vi "chooseKickTo.vi"(0 "KickToSkill in":refnum<class "KickToSkill.lvclass">, 1 "Game in":refnum<class "Game.lvclass">, 8 "Robot":refnum<class "Robot.lvclass">, 9 "KickForce 0?":bool, 10 "use criteria?":bool=TRUE, 11 "ForceInGame":bool, 12 "BadDribblerIDs":i32[](array[numeric]), 13 "pass?":bool, 15 "firstCall":bool, 16 "ChipKickInEnemyField":bool, 17 "Target":dbl[](array[numeric])) -> (20 "Game out":refnum<class "Game.lvclass">, 21 "Robot out":refnum<class "Robot.lvclass">)   [LabVIEW 2020, in "ShootTactic.lvclass"]
uses:
  ShootTactic.lvclass
  KickToSkill_class/KickToSkill.lvclass
  Robot_class/robotKickToStates.ctl
  Robot_class/Robot.lvclass
  Game_class/Game.lvclass
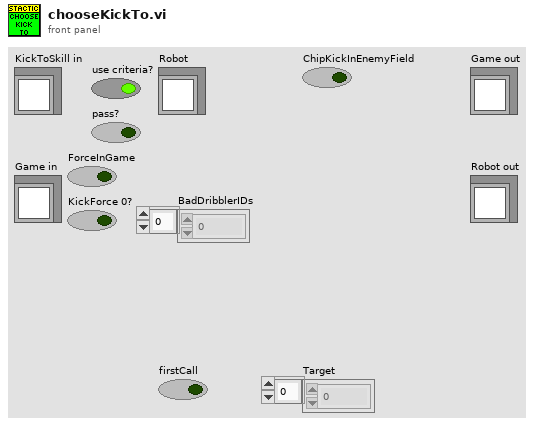
[diagram p1: front panel]
types:
  T1 = typedef "robotKickToStates.ctl" = enum16{"shootFromDirect", "avoidCollideBall", "goToBackBall", "none", "walk", "turn", "oldKickToShoot", "oldKickToGoToBackBall", "shoot"}
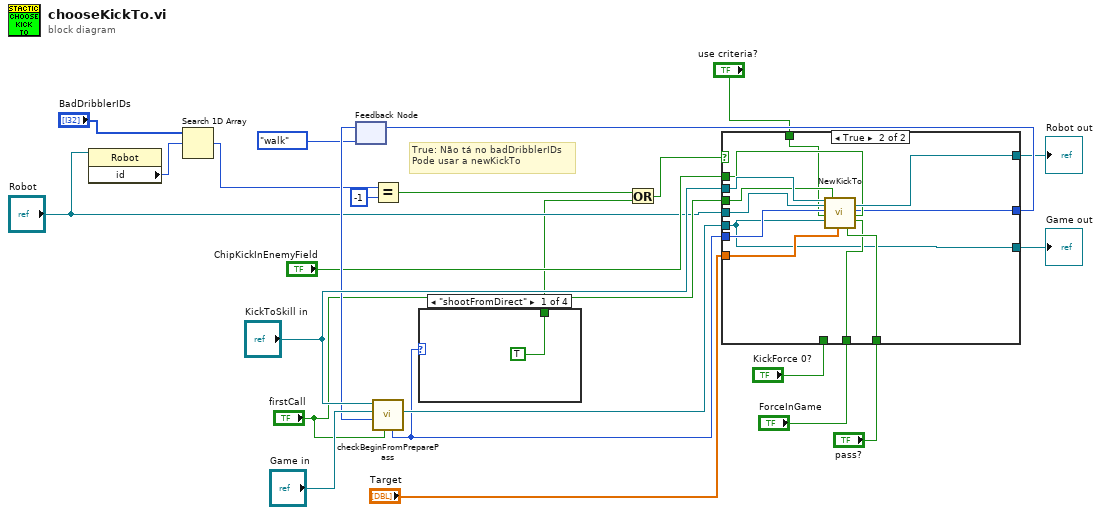
[diagram p0: block diagram]
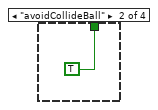
[diagram p2: hidden frame]
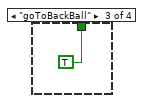
[diagram p3: hidden frame]
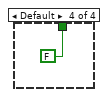
[diagram p4: hidden frame]
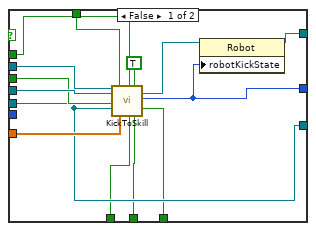
[diagram p5: hidden frame]
diagram:
  # "True: Não tá no badDribblerIDs\nPode usar a newKickTo"
  n1 = property class="Robot"(reference="Robot") -> ("id"=w7:i32)  [unwired: 1 in, 2 out]
  n2 = Search 1D Array(1D array="BadDribblerIDs", element=w7) -> (index of element=w6:i32)  [unwired: 1 in]
  n3 = feedback #1(robotKickToStates."walk" ("robotKickState")) -> (w20:T1)
  n4 = Equal?(x=w6, y=-1) -> (x = y?=w4:bool)
  n5 = call "checkBeginFromPreparePass.vi"("firstCall?"="firstCall", "robotKickState in"=w20, "Game in"="Game in", "KickToSkill in"="KickToSkill in") -> ("Game out"=w23:refnum<class "Game.lvclass">, "state out"=w3:T1)  [unwired: 3 in, 3 out]
  n6 = case shown="\"shootFromDirect\"" w3 {
    tunnel: [TRUE TRUE TRUE FALSE] -> w2
    frame "shootFromDirect" {
    }
    frame "avoidCollideBall" {
    }
    frame "goToBackBall" {
    }
    frame Default {
    }
  }
  n7 = Or(x=w4, y=w2) -> (x .or. y?=w5:bool)
  n8 = case shown="True" w5 {
    tunnel: "KickToSkill in" -> [w38 w54]
    tunnel: [w31 w53] -> w14
    tunnel: "Robot" -> [w42 w52]
    tunnel: "Target" -> [w40 w51]
    tunnel: w23 -> [w39 w43]
    tunnel: "firstCall" -> [w41 w50]
    tunnel: [w39 w43] -> w16
    tunnel: "ChipKickInEnemyField" -> [w37 w49]
    tunnel: w3 -> [_ w48]
    tunnel: [w30 w47] -> w24
    tunnel: "pass?" -> [w36 w45]
    tunnel: "ForceInGame" -> [w35 w44]
    tunnel: "KickForce 0?" -> [w34 _]
    tunnel: "use criteria?" -> [w33 w46]
    frame False {
      n9 = call "KickToSkill.vi"("KickToSkill in"=w38, "Robot"=w42, "firstCall?"=w41, "Game"=w39, "use criteria?"=w33, "Target"=w40, "chipKick ?"=w37, "KickForce 0?"=w34, "WeakKick"=TRUE, "ForceInGame"=w35, "pass?"=w36) -> ("Robot out"=w32:refnum<class "Robot.lvclass">, "robotKickState out"=w30:T1)  [unwired: 5 in, 2 out]
      n10 = property class="Robot"(reference=w32, "robotKickState"=w30) -> (reference out=w31:refnum<class "Robot.lvclass">)  [unwired: 1 in, 1 out]
    }
    frame True {
      n11 = call "NewKickTo.vi"("KickToSkill in"=w54, "Robot"=w52, "State in"=w48, "use criteria?"=w46, "Game"=w43, "firstCall?"=w50, "Target"=w51, "pass?"=w45, "chipKick ?"=w49, "ForceInGame"=w44) -> ("Robot out"=w53:refnum<class "Robot.lvclass">, "State out"=w47:T1)  [unwired: 6 in, 2 out]
    }
  }
  "Game out" <- w16
  "Robot out" <- w14
  n12 = feedback-in #1(w24) -> ()
